vi "TagDB_Find Names.vi"(8 "error in (no error)":errorcluster, 10 "RegExp":string, 11 "DB Ref":T1) -> (0 "error out":errorcluster, 1 "names":string[](array[string]), 3 "DB Ref(dup)":T1)   [LabVIEW 2017, in "TagDB.lvlib"]
doc: "[Covers: REQ_API_Value_NAME]"
uses:
  TagDB.lvlib
  Typedef/TagDB.ctl
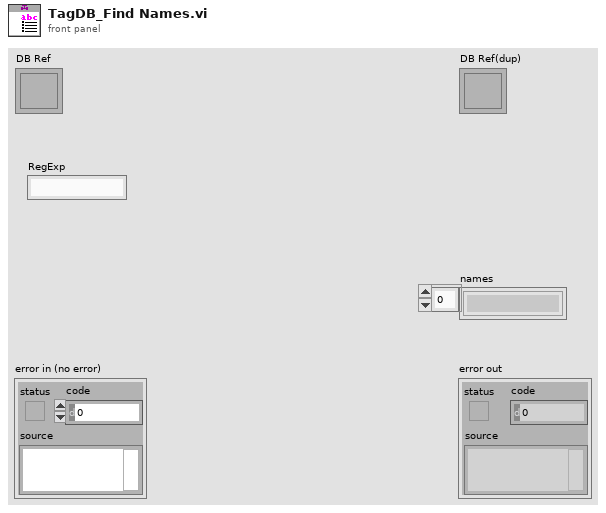
[diagram p1: front panel]
types:
  T1 = typedef "TagDB.lvlib/TagDB.ctl" = refnum<k1>
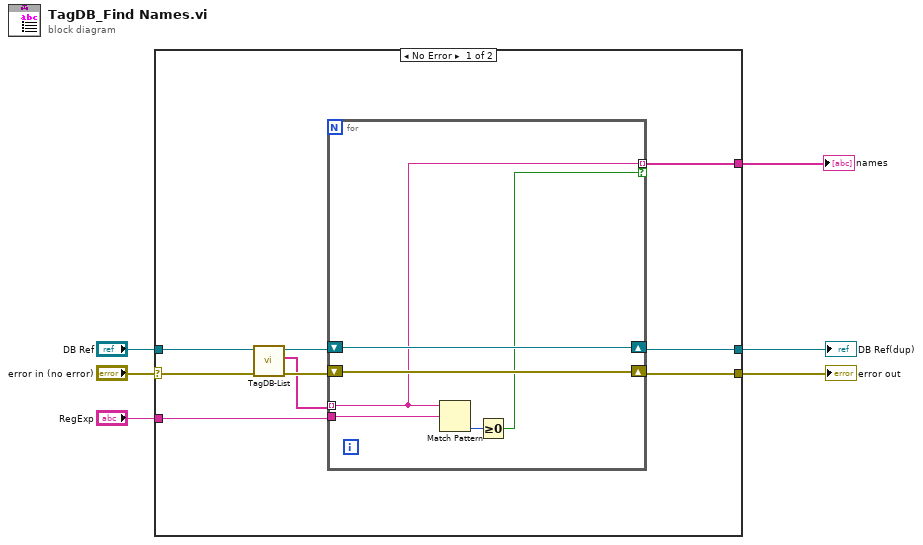
[diagram p0: block diagram]
diagram:
  n1 = case shown="No Error" "error in (no error)" {
    selector: "error in (no error)" -> [w13 w23]
    tunnel: [w10 w23] -> w5
    tunnel: [w15 w22] -> w3
    tunnel: "DB Ref" -> [w12 w22]
    tunnel: "RegExp" -> [w11 _]
    tunnel: [w14 _] -> w1
    frame No Error {
      n2 = call "TagDB-List.vi"("error in (no error)"=w13, "TagDB"=w12) -> ("error out"=w8:errorcluster, "names"=w7:string[], "TagDB(dup)"=w9:T1)  [unwired: 6 in, 1 out]
      n3 = for {
        tunnel: w11 -> [w19]
        shift-right: [w21] -> w15
        shift-left: w9 -> [w21]
        shift-right: [w20] -> w10
        shift-left: w8 -> [w20]
        tunnel: w7 -> [w18] mode=indexing
        tunnel: [w18] -> w14 mode=indexing if=w17
        n4 = Match Pattern(string=w18, regular expression=w19) -> (offset past match=w16:i32)  [unwired: 1 in, 3 out]
        n5 = Greater Or Equal To 0?(x=w16) -> (x >= 0?=w17:bool)
      }
    }
    frame Error {
    }
  }
  "error out" <- w5
  "DB Ref(dup)" <- w3
  "names" <- w1
